vi "Set Configuration.vi"(8 "error in (no error)":errorcluster, 11 "Input Signal in":refnum<class "Input Signal.lvclass">) -> (0 "error out":errorcluster, 3 "Input Signal out":refnum<class "Input Signal.lvclass">)   [LabVIEW 2015, in "Input Signal.lvclass"]
uses:
  Input Signal.lvclass
  IO Class/Direction.ctl
  IO Class/IO Class.lvclass
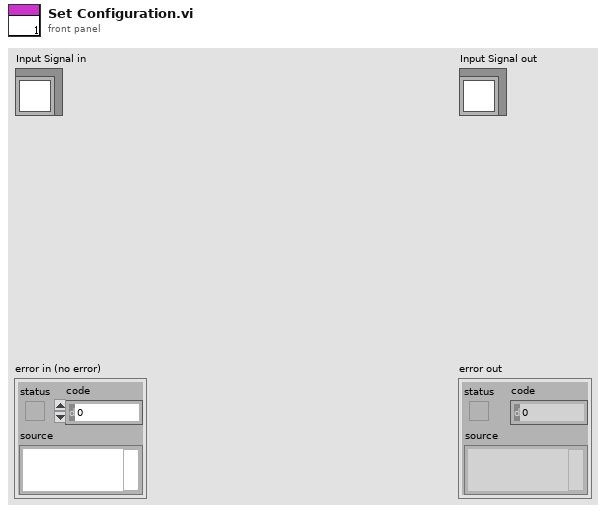
[diagram p1: front panel]
types:
  T1 = typedef "IO Class.lvclass/Direction.ctl" = cluster{"Direction":string}
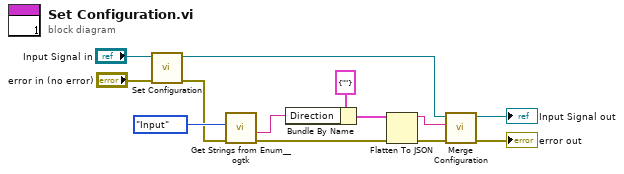
[diagram p0: block diagram]
diagram:
  n1 = call-parent "Set Configuration.vi"("error in (no error)"="error in (no error)", "IO Class in"="Input Signal in") -> ("error out"=w6:errorcluster, "IO Class out"=w5:refnum<class "Input Signal.lvclass">)  [unwired: 8 in]
  n2 = call <userlib>:"Get Strings from Enum__ogtk.vi"("error in (no error)"=w6, "Enum"=enum16{"Input", "Output"}."Input" ("Direction")) -> ("error out"=w9:errorcluster, "String Value"=w10:string)  [unwired: 6 in, 2 out]
  n3 = Bundle By Name(cluster=T1 {"Direction"=""} ("Cluster"), "Direction"=w10) -> (w8:T1)
  n4 = Flatten To JSON(anything=w8, error in (no error)=w9) -> (JSON string=w2:string, 11:w7:errorcluster)  [unwired: 1 in]
  n5 = call "Merge Configuration.vi"("error in (no error)"=w7, "Additional Configuration"=w2, "IO Class in"=w5) -> ("error out"=→"error out":errorcluster, "IO Class out"=→"Input Signal out":refnum<class "Input Signal.lvclass">)  [unwired: 7 in]
